vi "ScanWhat.vi"(10 "DyeLaser":T2={"Scan.Start (cm-1)"=15000.0, "Scan.Stop (cm-1)"=15050.0, "Scan.step (cm-1)"=0.2, "dye laser port"="", "Laser"=enum."Syrah", "NSteps"=251, "CurrentStep"=75, "Current.cm-1"=15015.0} {"Current.cm-1" format="%.2f"}, 11 "Camera":T1={"Gate.Delay"=0, "Delay.Step"=0, "Gate.Duration"=150000, "#Accum"=10, "SetpointTemp"=-30, "Last Temp"=6, "Current Temp"=4}) -> (0 "ScanWhat?":enum16{"nothing", "laser", "delay"}(ring), 2 "DyeLaser out":T2={"Scan.Start (cm-1)"=15000.0, "Scan.Stop (cm-1)"=15050.0, "Scan.step (cm-1)"=0.2, "dye laser port"="", "Laser"=enum."Syrah", "NSteps"=251, "CurrentStep"=75, "Current.cm-1"=15015.0} {"Current.cm-1" format="%.2f"}, 3 "Camera out":T1={"Gate.Delay"=0, "Delay.Step"=0, "Gate.Duration"=150000, "#Accum"=10, "SetpointTemp"=-30, "Last Temp"=6, "Current Temp"=4})   [LabVIEW 2022 SP3]
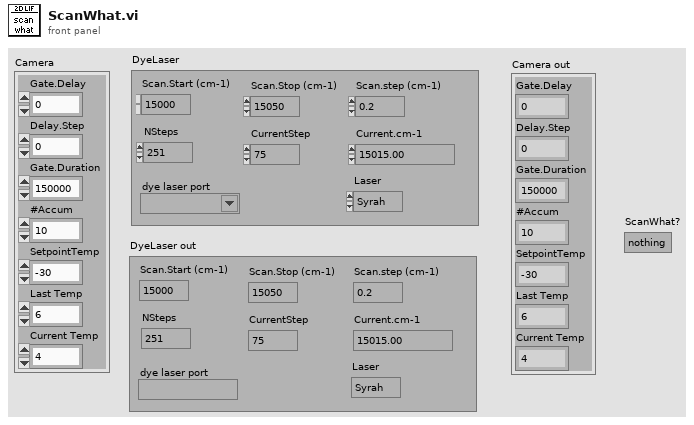
[diagram p1: front panel]
types:
  T1 = cluster{"Gate.Delay":u64, "Delay.Step":u64, "Gate.Duration":u64, "#Accum":i32, "SetpointTemp":i32, "Last Temp":i32, "Current Temp":i32}
  T2 = cluster{"Scan.Start (cm-1)":dbl, "Scan.Stop (cm-1)":dbl, "Scan.step (cm-1)":dbl, "dye laser port":refnum<visa-resource-name>, "Laser":enum16{"Syrah", "Hyperdye"}, "NSteps":i32, "CurrentStep":i32, "Current.cm-1":dbl}
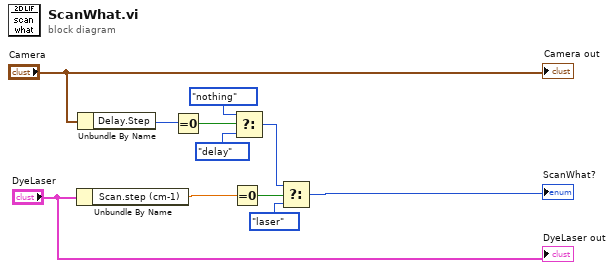
[diagram p0: block diagram]
diagram:
  n1 = Unbundle By Name("DyeLaser") -> ("Scan.step (cm-1)"=w10:dbl)
  n2 = Unbundle By Name("Camera") -> ("Delay.Step"=w2:u64)
  n3 = Equal To 0?(x=w2) -> (x = 0?=w9:bool)
  n4 = Equal To 0?(x=w10) -> (x = 0?=w6:bool)
  n5 = Select(t=enum16{"nothing", "laser", "delay"}."nothing" ("ScanWhat?"), s=w9, f=enum16{"nothing", "laser", "delay"}."delay" ("ScanWhat?")) -> (s? t:f=w4:enum16{"nothing", "laser", "delay"})
  n6 = Select(t=w4, s=w6, f=enum16{"nothing", "laser", "delay"}."laser" ("ScanWhat?")) -> (s? t:f=→"ScanWhat?":enum16{"nothing", "laser", "delay"})
  "DyeLaser out" <- "DyeLaser"
  "Camera out" <- "Camera"
